vi "Set View Control Reference.vi"(8 "error in (no error)":errorcluster, 10 "View Control":refnum<vi>, 11 "Chronological List in":refnum<class "Chronological List.lvclass">) -> (0 "error out":errorcluster, 3 "Chronological List out":refnum<class "Chronological List.lvclass">)   [LabVIEW 2020, in "Chronological List.lvclass"]
uses:
  Chronological List.lvclass
  <vilib>/Utility/miscctls.llb/LVRowAndColumnUnsignedTypeDef.ctl
  Chronological List.lvclass/Chronological List.ctl
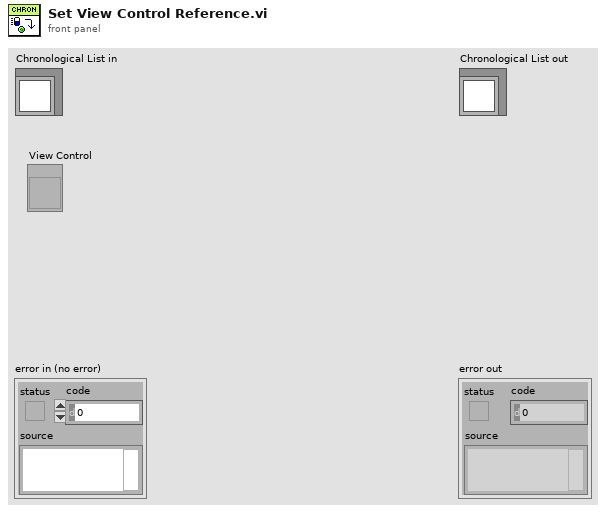
[diagram p1: front panel]
types:
  T1 = typedef "LVRowAndColumnUnsignedTypeDef.ctl" = cluster{"Row":u32, "Column":u32}
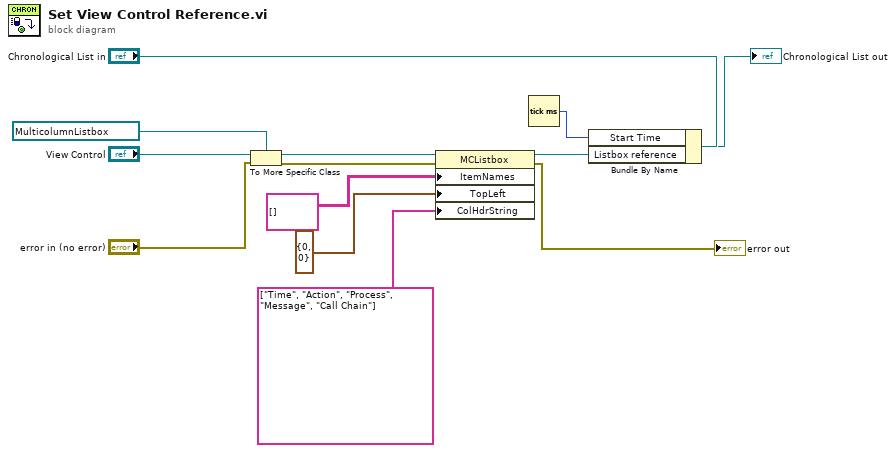
[diagram p0: block diagram]
diagram:
  n1 = To More Specific Class(target class=refnum<vi> refnum ("Listbox reference"), reference="View Control", error in="error in (no error)") -> (specific class reference=w8:refnum<vi>, error out=w5:errorcluster)
  n2 = property on="Property Node" class="MCListbox"(reference=w8, error in=w5, "ItemNames"=string[][] [] ("Item Names"), "TopLeft"=T1 {"Row"=0, "Column"=0} ("Top Left Visible Cell"), "ColHdrString"=string[] ["Time", "Action", "Process", "Message", "Call Chain"] ("Column Header Strings[]")) -> (reference out=w7:refnum<vi>, error out=→"error out":errorcluster)
  n3 = Tick Count (ms)() -> (millisecond timer value=w1:u32)
  n4 = Bundle By Name(cluster="Chronological List in", "Start Time"=w1, "Listbox reference"=w7) -> (→"Chronological List out":refnum<class "Chronological List.lvclass">)
